vi "PID.vi"() -> ()   [LabVIEW 2017]
panel:
  out "syg  wej":dbl(graph)
  out "syg wyj":dbl(graph)
  in  "device name":tag="Dev1"
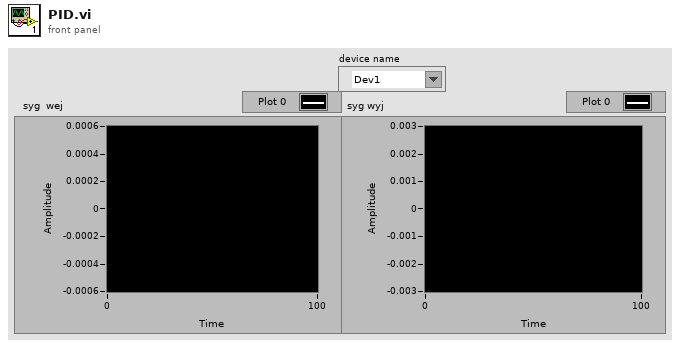
[diagram p1: front panel]
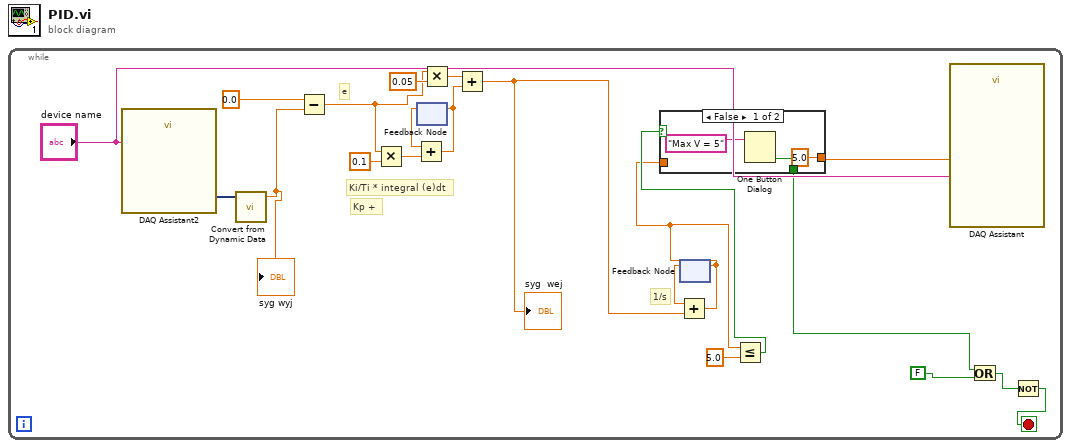
[diagram p0: block diagram]
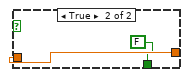
[diagram p2: hidden frame]
diagram:
  n1 = while {
    stop <- w3 stop-if-true
    # "1/s"
    # "Kp +"
    # "Ki/Ti * integral (e)dt"
    # "e"
    n2 = call "DAQ Assistant2"("device name"="device name") -> ("data"=w18:dynamicdata)  [unwired: 16 in, 2 out]
    n3 = call "Convert from Dynamic Data"("Dynamic Data Type"=w18) -> ("Scalar"=w17:dbl)  [unwired: 3 in]
    "syg wyj" <- w17
    n4 = Subtract(x=0.0, y=w17) -> (x-y=w10:dbl)
    n5 = Multiply(x=w10, y=0.1) -> (x*y=w15:dbl)
    n6 = feedback #1() -> (w16:dbl)  [unwired: 1 in]
    n7 = Add(x=w16, y=w15) -> (x+y=w13:dbl)
    n8 = feedback-in #1(w13) -> ()
    n9 = Multiply(x=w10, y=0.05) -> (x*y=w12:dbl)
    n10 = Add(x=w12, y=w13) -> (x+y=w9:dbl)
    "syg  wej" <- w9
    n11 = feedback #2() -> (w19:dbl)  [unwired: 1 in]
    n12 = Add(x=w19, y=w9) -> (x+y=w5:dbl)
    n13 = feedback-in #2(w5) -> ()
    n14 = Less Or Equal?(x=w5, y=5.0) -> (x <= y?=w7:bool)
    n15 = case shown="False" w7 {
      tunnel: [5.0 w26] -> w6
      tunnel: w5 -> [_ w26]
      tunnel: [w23 FALSE] -> w1
      frame False {
        n16 = One Button Dialog(message="Max V = 5") -> (true=w23:bool)  [unwired: 1 in]
      }
      frame True {
      }
    }
    n17 = call "DAQ Assistant"("data"=w6, "device name"="device name") -> ()  [unwired: 16 in, 2 out]
    n18 = Or(x=w1, y=FALSE) -> (x .or. y?=w4:bool)
    n19 = Not(x=w4) -> (.not. x?=w3:bool)
  }
